vi "problem_2_part3.vi"() -> ()   [LabVIEW 2020]
panel:
  out "Fahrenheit":dbl(slide) scale=0.0..100.0
  out "Celsius":dbl(slide) scale=0.0..100.0
  in  "Kelvins":dbl
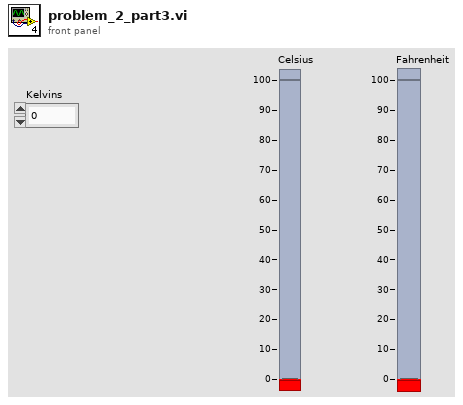
[diagram p1: front panel]
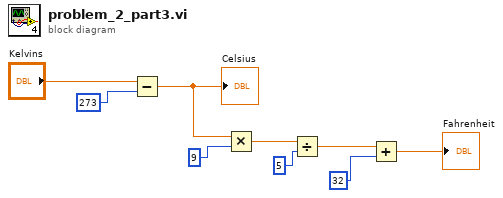
[diagram p0: block diagram]
diagram:
  n1 = Subtract(x="Kelvins", y=273) -> (x-y=w6:dbl)
  "Celsius" <- w6
  n2 = Multiply(x=w6, y=9) -> (x*y=w5:dbl)
  n3 = Divide(x=w5, y=5) -> (x/y=w3:dbl)
  n4 = Add(x=w3, y=32) -> (x+y=→"Fahrenheit":dbl)
